vi "AuMT8852B Inquiry.vi"(7 "Start/Stop (Start)":enum16{"Start", "Stop"}(ring), 8 "error in (no error)":errorcluster, 11 "VISA session":refnum<visa-resource-name>) -> (0 "error out":errorcluster, 2 "error code":i32, 3 "VISA session out":refnum<visa-resource-name>)   [LabVIEW 2017]
doc: "Anritsu MT8852B Bluetooth Tester\n\nStarts or stops the inquiry defined by the inquiry configuration functions.\n\nINPUTS\nStart/Stop - whether to perform or cancel an inquiry."
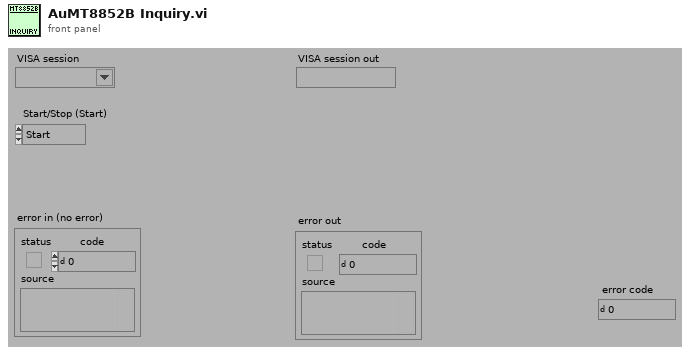
[diagram p1: front panel]
types:
  T1 = enum16{"Simulate", "Range check", "Cache", "Query instrument status"}
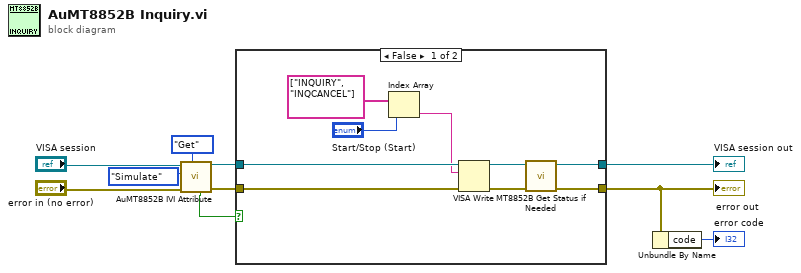
[diagram p0: block diagram]
diagram:
  n1 = call <instrlib>:"AuMT8852B IVI Attribute.vi"("Set/Get (Set)"=enum16{"Set", "Get"}."Get", "error in (no error)"="error in (no error)", "Flag (Simulate)"=T1."Simulate", "VISA session"="VISA session") -> ("error out"=w6:errorcluster, "VISA session out"=w7:refnum<visa-resource-name>, "Value out"=w3:bool)  [unwired: 5 in]
  n2 = case shown="False" w3 {
    tunnel: [w16 w20] -> w10
    tunnel: [w15 w21] -> w1
    tunnel: w7 -> [w19 w20]
    tunnel: w6 -> [w18 w21]
    frame False {
      n3 = Index Array(array=string[] ["INQUIRY", "INQCANCEL"] ("Array Constant"), index="Start/Stop (Start)") -> (element=w12:string)
      n4 = VISA Write(VISA resource name=w19, write buffer=w12, error in (no error)=w18) -> (VISA resource name out=w17:refnum<visa-resource-name>, error out=w14:errorcluster)  [unwired: 1 out]
      n5 = call <instrlib>:"MT8852B Get Status if Needed.vi"("error in (no error)"=w14, "VISA session"=w17) -> ("error out"=w15:errorcluster, "VISA session out"=w16:refnum<visa-resource-name>)  [unwired: 8 in]
    }
    frame True {
    }
  }
  "VISA session out" <- w10
  "error out" <- w1
  n6 = Unbundle By Name(w1) -> ("code"=→"error code":i32)
